vi "New File.vi"(8 "error in (no error)":errorcluster, 11 "Refnum":refnum<k7>) -> (0 "error out":errorcluster, 2 "File refnum":refnum<k7>, 3 "App refnum out":refnum<k7>)   [LabVIEW 2020, in "lvpptx.lvlib"]
uses:
  lvpptx.lvlib
panel:
  # "Create a new .pptx file"
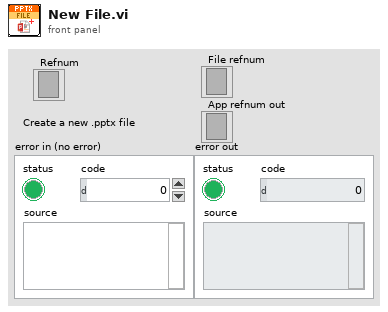
[diagram p1: front panel]
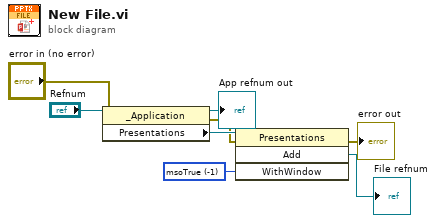
[diagram p0: block diagram]
diagram:
  w6 = -1 items=["msoTrue"=-1, "msoFalse"=0, "msoCTrue"=1, "msoTriStateToggle"=-3, "msoTriStateMixed"=-2] ("WithWindow")
  n1 = property class="_Application"(reference="Refnum", error in="error in (no error)") -> (reference out=→"App refnum out":refnum<k7>, error out=w5:errorcluster, "Presentations"=w7:refnum<k7>)
  n2 = invoke class="Presentations" method="Add"(reference=w7, error in=w5, "WithWindow"=w6) -> (error out=→"error out":errorcluster, "Add"=→"File refnum":refnum<k7>)  [unwired: 1 in, 2 out]
